vi "Weight--constant.vi"() -> (3 "Weight":i32)   [LabVIEW 2020, in "Performance Monitor UI.lvlib" / "Configuration.lvlib"]
doc: "The relative weight of this configuration page. The lower the value, the higher it will appear in the list in the Configuration UIs.\n_____\nBased on DCFG Project Template 1.0.0.21.\n____\nPeloton Config 1.0.0.2\nCopyright (c) 2022, Peloton"
uses:
  Configuration.lvlib
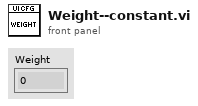
[diagram p1: front panel]
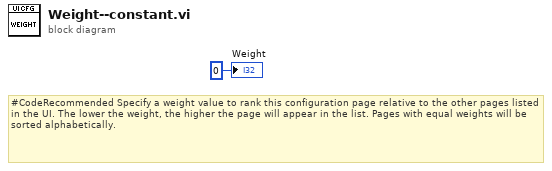
[diagram p0: block diagram]
diagram:
  # "#CodeRecommended Specify a weight value to rank this configuration page relative to the other pages listed in the UI. The lower the weight, the higher the page will appear in the list. Pages with equal weights will be sorted alphabetically."
  "Weight" <- 0 ("Weight")
